vi "Get Timestamp from UUID-value Lists.vi"(10 "UUIDs":string[](array[string]), 11 "Values":dbl[](array[numeric])) -> (0 "error out":errorcluster, 3 "time stamp":timestamp)   [LabVIEW 2020]
uses:
  <vilib>/Utility/miscctls.llb/LVDateTimeRec.ctl
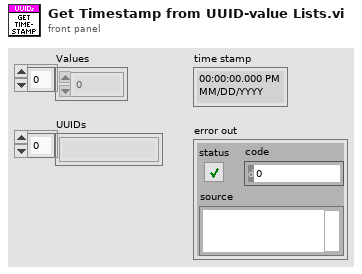
[diagram p1: front panel]
types:
  T1 = typedef "LVDateTimeRec.ctl" = cluster{"fractional second":dbl, "second":i32, "minute":i32, "hour":i32, "day of month":i32, "month":i32, "year":i32, "day of week":i32, "day of year":i32, "DST":i32}
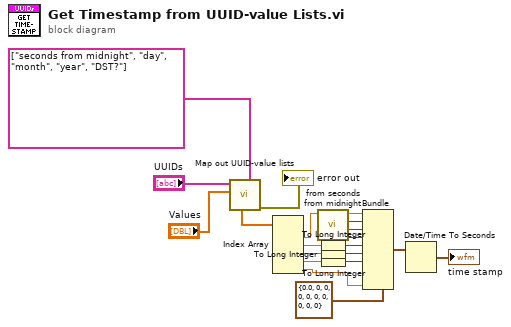
[diagram p0: block diagram]
diagram:
  n1 = call "Map out UUID-value lists.vi"("UUIDs to extract"=string[] ["seconds from midnight", "day", "month", "year", "DST?"], "values in"="Values", "UUIDs in"="UUIDs") -> ("error out"=→"error out":errorcluster, "values extracted"=w15:dbl[])  [unwired: 4 in, 3 out]
  n2 = Index Array(array=w15) -> (element #1=w7:dbl, element #2=w8:dbl, element #3=w9:dbl, element #4=w10:dbl, element #5=w18:dbl)  [unwired: 5 in]
  n3 = call "from seconds from midnight.vi"("seconds from 00:00"=w7) -> ("hour"=w5:i32, "minute"=w4:i32, "second"=w3:i32, "fractional second"=w2:dbl)  [unwired: 7 in]
  n4 = To Long Integer(number=w8) -> (32bit integer=w11:i32)
  n5 = To Long Integer(number=w9) -> (32bit integer=w12:i32)
  n6 = To Long Integer(number=w10) -> (32bit integer=w13:i32)
  n7 = Bundle(cluster=T1 {"fractional second"=0.0, "second"=0, "minute"=0, "hour"=0, "day of month"=0, "month"=0, "year"=0, "day of week"=0, "day of year"=0, "DST"=0} ("date time rec"), "fractional second"=w2, "second"=w3, "minute"=w4, "hour"=w5, "day of month"=w11, "month"=w12, "year"=w13, "DST"=w18) -> (w1:T1)  [unwired: 2 in]
  n8 = Date/Time To Seconds(2:w1) -> (0:→"time stamp":timestamp)  [unwired: 1 in]
